vi "Import Export - Temp SDF Load EC CD from XML.vi"(8 "Error In":errorcluster, 10 "Cfiguration File Path":path, 11 "Temp SDF Refnum In":refnum<k24>) -> (0 "Error Out":errorcluster, 2 "Temp EC CD Item Ref":T1 format="%.0x", 3 "Temp SDF Refnum Out":refnum<k24>)   [LabVIEW 2017, in "Scan Engine Custom Device.lvlib"]
uses:
  Scan Engine Custom Device.lvlib
  NationalInstruments.VeriStand.SystemDefinitionAPI
  <vilib>/NI Veristand/Custom Device API/Custom Device Item Ref.ctl
  <vilib>/NI/NI VeriStand Advanced SysDef API/_Types/SysDef.Export.ctl
  <vilib>/NI/NI VeriStand Advanced SysDef API/_Types/TreeItem.ctl
  <vilib>/NI/NI VeriStand Advanced SysDef API/_Types/TreeItem.Info.ctl
  <vilib>/NI Veristand/Custom Device API/Custom Device Channel.ctl
  <vilib>/NI Veristand/Custom Device API/Custom Device Channel Type.ctl
  <vilib>/NI Veristand/Custom Device API/Custom Device Waveform.ctl
  <vilib>/NI Veristand/Custom Device API/Custom Device Waveform DataType.ctl
  <vilib>/NI/NI VeriStand Advanced SysDef API/_Types/TreeItem.Property.ctl
  Globals/Scan Engine GUIDs.vi
  <vilib>/NI/NI VeriStand Custom Device Import and Export Tool/ImportExport.lvlib
  <vilib>/NI/NI VeriStand Advanced SysDef API/SysDef API/Advanced System Definition.lvlib
  <vilib>/NI Veristand/Custom Device API/Custom Device API.lvlib
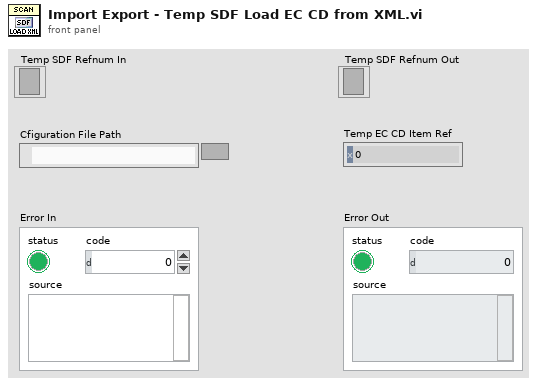
[diagram p1: front panel]
types:
  T1 = typedef "Custom Device API.lvlib/Custom Device Item Ref.ctl" = u64
  T2 = cluster{"Creator":string, "Target Name":string, "Target Type":string, "IP Address":string}
  T3 = typedef "Advanced System Definition.lvlib/SysDef.Export.ctl" = cluster{"Version":string, "Tree":T4[]}
  T4 = typedef "Advanced System Definition.lvlib/TreeItem.ctl" = cluster{"Item Info":T5, "Parent Path":string[], "Properties":T10[]}
  T5 = typedef "Advanced System Definition.lvlib/TreeItem.Info.ctl" = cluster{"Name":string, "Description":string, "GUID":string, "Is Channel":bool, "Channel":T6, "Is Waveform":bool, "Waveform":T8}
  T6 = typedef "Custom Device API.lvlib/Custom Device Channel.ctl" = cluster{"Type":T7, "Units":string, "Default Value":dbl, "Faultable":bool, "Scalable":bool}
  T7 = typedef "Custom Device API.lvlib/Custom Device Channel Type.ctl" = enum16{"Input", "Output"}
  T8 = typedef "Custom Device API.lvlib/Custom Device Waveform.ctl" = cluster{"Data Type":T9, "Units":string}
  T9 = typedef "Custom Device API.lvlib/Custom Device Waveform DataType.ctl" = enum16{"Double", "Complex Double"}
  T10 = typedef "Advanced System Definition.lvlib/TreeItem.Property.ctl" = cluster{"Name":string, "Type":i32, "Value":variant}
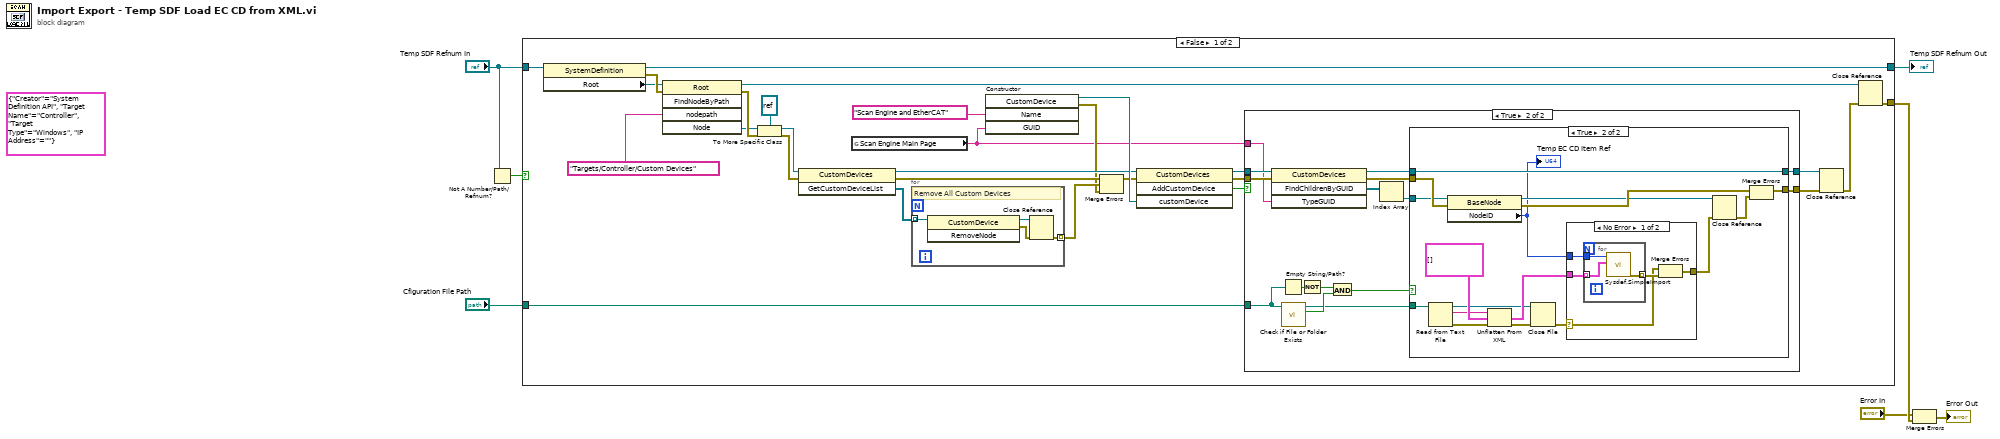
[diagram p0: block diagram]
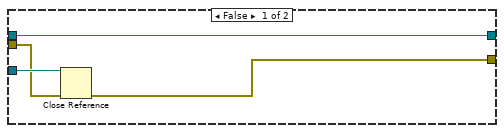
[diagram p3: hidden frame]
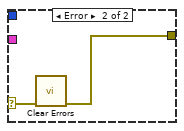
[diagram p4: hidden frame]
diagram:
  (unwired) T2 {"Creator"="System Definition API", "Target Name"="Controller", "Target Type"="Windows", "IP Address"=""} ("New SDF Information")
  n1 = Not A Number/Path/Refnum?(number/path/refnum="Temp SDF Refnum In") -> (NaN/Path/Refnum?=w3:bool)
  n2 = case shown="False" w3 {
    tunnel: [w34 _] -> w7
    tunnel: [w23 w88] -> w4
    tunnel: "Temp SDF Refnum In" -> [w22 w88]
    tunnel: "Cfiguration File Path" -> [w20 _]
    frame False {
      n3 = property class="SystemDefinition"(reference=w22) -> (reference out=w23:refnum<k24>, error out=w33:errorcluster, "Root"=w24:refnum<k24>)  [unwired: 1 in]
      n4 = invoke class="Root" method="FindNodeByPath"(reference=w24, error in=w33, "nodepath"="Targets/Controller/Custom Devices") -> (reference out=w32:refnum<k24>, error out=w31:errorcluster, "Node"=w30:refnum<k24>)  [unwired: 2 in, 2 out]
      n5 = To More Specific Class(target class=refnum<k24> refnum ("reference"), reference=w30, error in=w31) -> (specific class reference=w16:refnum<k24>, error out=w26:errorcluster)
      n6 = invoke class="CustomDevices" method="GetCustomDeviceList"(reference=w16, error in=w26) -> (reference out=w14:refnum<k24>, error out=w21:errorcluster, "GetCustomDeviceList"=w28:refnum<k24>[])  [unwired: 1 in]
      n7 = global read "Scan Engine GUIDs.vi" "Scan Engine Main Page"() -> (w9:string)
      n8 = for "Remove All Custom Devices" {
        tunnel: w28 -> [w86] mode=indexing
        tunnel: [w87] -> w27 mode=indexing
        # "Remove All Custom Devices"
        n9 = invoke class="CustomDevice" method="RemoveNode"(reference=w86) -> (reference out=w84:refnum<k24>, error out=w85:errorcluster)  [unwired: 2 in, 1 out]
        n10 = Close Reference(reference=w84, error in (no error)=w85) -> (error out=w87:errorcluster)
      }
      n11 = constructor class="CustomDevice"("Name"="Scan Engine and EtherCAT", "GUID"=w9) -> (reference out=w15:refnum<k24>, error out=w12:errorcluster)  [unwired: 3 in, 3 out]
      n12 = Merge Errors(w21, w27, w12) -> (w13:errorcluster)
      n13 = invoke class="CustomDevices" method="AddCustomDevice"(reference=w14, error in=w13, "customDevice"=w15) -> (reference out=w11:refnum<k24>, error out=w10:errorcluster, "AddCustomDevice"=w8:bool)  [unwired: 1 in, 1 out]
      n14 = case shown="True" w8 {
        tunnel: w20 -> [_ w49]
        tunnel: [w37 w47] -> w19
        tunnel: [w36 w46] -> w18
        tunnel: w11 -> [w37 w45]
        tunnel: w10 -> [w36 w43]
        tunnel: w9 -> [_ w41]
        frame False {
        }
        frame True {
          n15 = invoke class="CustomDevices" method="FindChildrenByGUID"(reference=w45, error in=w43, "TypeGUID"=w41) -> (reference out=w44:refnum<k24>, error out=w42:errorcluster, "FindChildrenByGUID"=w40:refnum<k24>[])  [unwired: 1 in, 1 out]
          n16 = Empty String/Path?(string/path=w49) -> (empty?=w52:bool)
          n17 = call <vilib>:"Check if File or Folder Exists.vi"("path"=w49) -> ("file or folder exists?"=w51:bool, "dup path"=w48:path)  [unwired: 8 in, 1 out]
          n18 = Not(x=w52) -> (.not. x?=w50:bool)
          n19 = And(x=w50, y=w51) -> (x .and. y?=w38:bool)
          n20 = Index Array(array=w40) -> (element=w39:refnum<k24>)  [unwired: 1 in]
          n21 = case shown="True" w38 {
            tunnel: w48 -> [_ w68]
            tunnel: w44 -> [w56 w58]
            tunnel: w42 -> [w54 w73]
            tunnel: [w56 w58] -> w47
            tunnel: [w53 w63] -> w46
            tunnel: w39 -> [w55 w62]
            frame False {
              n22 = Close Reference(reference=w55, error in (no error)=w54) -> (error out=w53:errorcluster)
            }
            frame True {
              n23 = Read from Text File(file (use dialog)=w68) -> (refnum out=w67:refnum<file>, text=w69:string, error out=w70:errorcluster)  [unwired: 3 in, 1 out]
              n24 = property class="BaseNode"(reference=w62, error in=w73) -> (reference out=w60:refnum<k24>, error out=w64:errorcluster, "NodeID"=w57:u64)
              "Temp EC CD Item Ref" <- w57
              n25 = Unflatten From XML(xml string=w69, type=T3[] [], error in (no error)=w70) -> (value=w71:T3[], error out=w66:errorcluster)
              n26 = Close File(refnum=w67, error in=w66) -> (error out=w65:errorcluster)  [unwired: 1 out]
              n27 = case shown="No Error" w65 {
                selector: w65 -> [w74 w83]
                tunnel: w71 -> [w78 _]
                tunnel: w57 -> [w77 _]
                tunnel: [w75 w82] -> w61
                frame No Error {
                  n28 = for {
                    tunnel: w78 -> [w81] mode=indexing
                    tunnel: w77 -> [w80]
                    tunnel: [w79] -> w76 mode=indexing
                    n29 = call <vilib>:"Sysdef.SimpleImport.vi"("SysDef"=w81, "NodeID"=w80) -> ("error out"=w79:errorcluster)  [unwired: 8 in, 1 out]
                  }
                  n30 = Merge Errors(w74, w76) -> (w75:errorcluster)
                }
                frame Error {
                  n31 = call <vilib>:"Clear Errors.vi"("error in (no error)"=w83) -> ("error out"=w82:errorcluster)  [unwired: 5 in, 1 out]
                }
              }
              n32 = Close Reference(reference=w60, error in (no error)=w61) -> (error out=w59:errorcluster)
              n33 = Merge Errors(w64, w59) -> (w63:errorcluster)
            }
          }
        }
      }
      n34 = Close Reference(reference=w19, error in (no error)=w18) -> (error out=w35:errorcluster)
      n35 = Close Reference(reference=w32, error in (no error)=w35) -> (error out=w34:errorcluster)
    }
    frame True {
    }
  }
  "Temp SDF Refnum Out" <- w4
  n36 = Merge Errors("Error In", w7) -> (→"Error Out":errorcluster)
